vi "Compare.vi"(8 "error in (no error)":errorcluster, 10 "Level":dbl, 11 "Aim Lower Threshold in":refnum<class "Aim Lower Threshold.lvclass">) -> (0 "error out":errorcluster, 2 "Color":u32(colorbox))   [LabVIEW 2021, in "Aim Lower Threshold.lvclass"]
uses:
  Aim Lower Threshold.lvclass
  Utilities/Colors.ctl
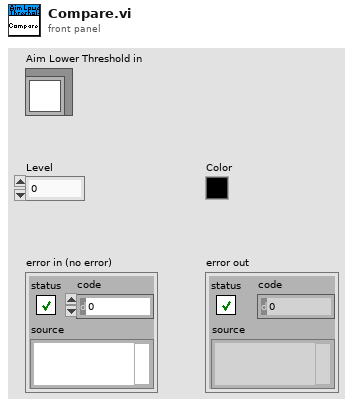
[diagram p1: front panel]
types:
  T1 = typedef "Colors.ctl" = cluster{"Green":u32, "Yellow":u32, "Red":u32}
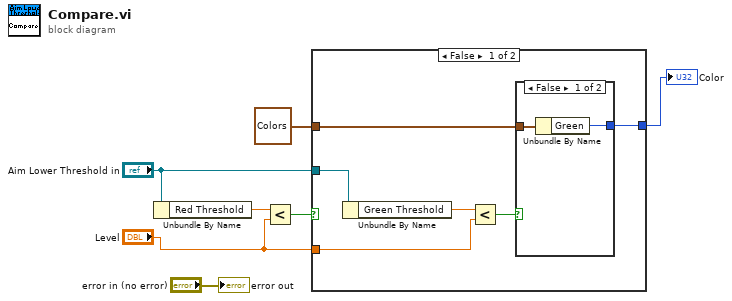
[diagram p0: block diagram]
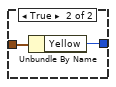
[diagram p2: hidden frame]
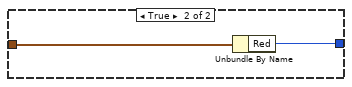
[diagram p3: hidden frame]
diagram:
  n1 = Unbundle By Name("Aim Lower Threshold in") -> ("Red Threshold"=w6:dbl)
  n2 = Less?(x=w6, y="Level") -> (x < y?=w7:bool)
  n3 = case shown="False" w7 {
    tunnel: [w13 w19] -> w4
    tunnel: "Level" -> [w11 _]
    tunnel: "Aim Lower Threshold in" -> [w10 _]
    tunnel: T1 {"Green"=65408, "Yellow"=16777088, "Red"=16744576} ("Colors") -> [w8 w18]
    frame False {
      n4 = Unbundle By Name(w10) -> ("Green Threshold"=w9:dbl)
      n5 = Less?(x=w9, y=w11) -> (x < y?=w12:bool)
      n6 = case shown="False" w12 {
        tunnel: [w15 w17] -> w13
        tunnel: w8 -> [w14 w16]
        frame False {
          n7 = Unbundle By Name(w14) -> ("Green"=w15:u32)
        }
        frame True {
          n8 = Unbundle By Name(w16) -> ("Yellow"=w17:u32)
        }
      }
    }
    frame True {
      n9 = Unbundle By Name(w18) -> ("Red"=w19:u32)
    }
  }
  "Color" <- w4
  "error out" <- "error in (no error)"
